vi "Obtain Timestamp.vi"(8 "error in (no error)":errorcluster, 11 "ControlRefnumArray":refnum<vi>[](array[refnum])) -> (0 "error out":errorcluster, 2 "Time Stamp":timestamp, 3 "Array":refnum<vi>[](array[refnum]))   [LabVIEW 2016, in "M1M3SupportEUI_Views.lvlib"]
uses:
  M1M3SupportEUI_Views.lvlib
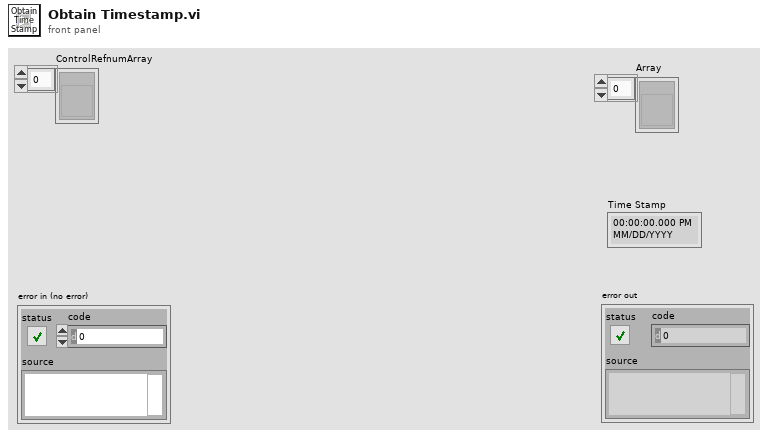
[diagram p1: front panel]
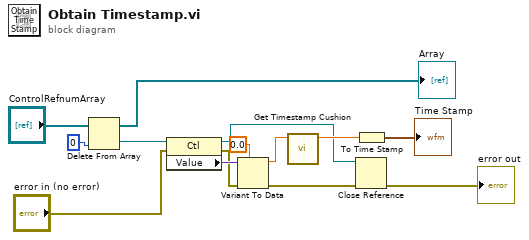
[diagram p0: block diagram]
diagram:
  n1 = Delete From Array(array="ControlRefnumArray", index=0) -> (deleted portion=w8:refnum<vi>, array with subset deleted=→"Array":refnum<vi>[])  [unwired: 1 in]
  n2 = property class="Ctl"(reference=w8, error in="error in (no error)") -> (reference out=w3:refnum<vi>, error out=w12:errorcluster, "Value"=w14:variant)
  n3 = Variant To Data(error in=w12, type=0.0, Variant=w14) -> (data=w5:dbl, error out=w6:errorcluster)
  n4 = call "Get Timestamp Cushion.vi"("DoubleTimestampRepresentation"=w5) -> ("TimestampCushion"=w4:dbl)  [unwired: 10 in]
  n5 = Close Reference(reference=w3, error in (no error)=w6) -> (error out=→"error out":errorcluster)
  n6 = To Time Stamp(1:w4) -> (0:→"Time Stamp":timestamp)
